vi "testExpressElapsedTime.vi"() -> ()   [LabVIEW 2014]
panel:
  out "Elapsed Time (s) 2":dbl caption="Verstrichene Zeit (s)"
  out "Elapsed Time (s)":dbl caption="Verstrichene Zeit (s)"
  in  "Stopp":bool
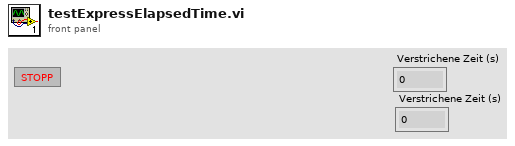
[diagram p1: front panel]
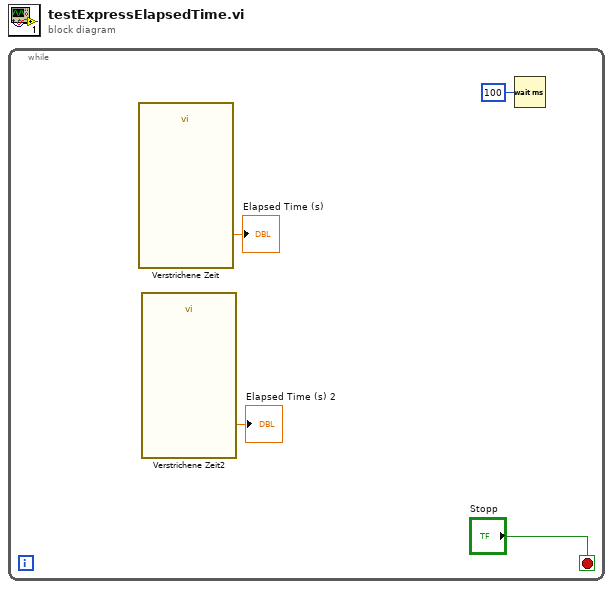
[diagram p0: block diagram]
diagram:
  n1 = while {
    stop <- "Stopp" stop-if-true
    n2 = call "Verstrichene Zeit"() -> ("Elapsed Time (s)"=→"Elapsed Time (s)":dbl)  [unwired: 12 in, 7 out]
    n3 = call "Verstrichene Zeit2"() -> ("Elapsed Time (s)"=→"Elapsed Time (s) 2":dbl)  [unwired: 12 in, 7 out]
    n4 = Wait (ms)(milliseconds to wait=u32 100 ("Zu wartende ms")) -> ()  [unwired: 1 out]
  }
